vi "EMV T7 Flow Conditions.vi"(4 "Detection Slope":dbl=0.2 format="%#_13g", 7 "Mixing Valve.Flow State (0x4009)":u8, 8 "error in (no error)":errorcluster, 10 "T7_DELTA_FLOW_THRESHOLD":dbl, 11 "T7 History":dbl[](array[numeric])) -> (0 "error out":errorcluster, 1 "PI Detect?":bool, 2 "T7 Detect?":bool, 3 "Flow Detect?":bool)   [LabVIEW 2020]
panel:
  out "Slope Chart":dbl(graph)
  in  "T7_DELTA_INDICATING_FLOW":dbl
  in  "Cold Water Supply Temperature":dbl
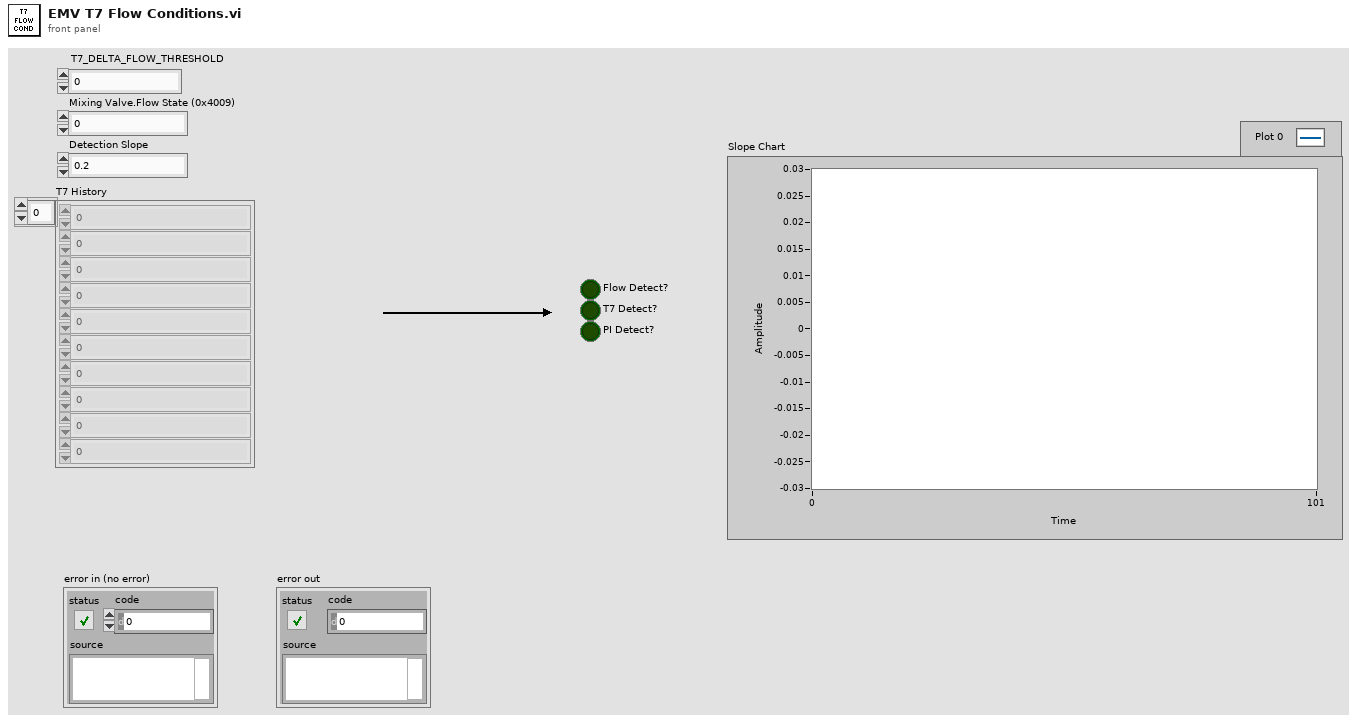
[diagram p1: front panel]
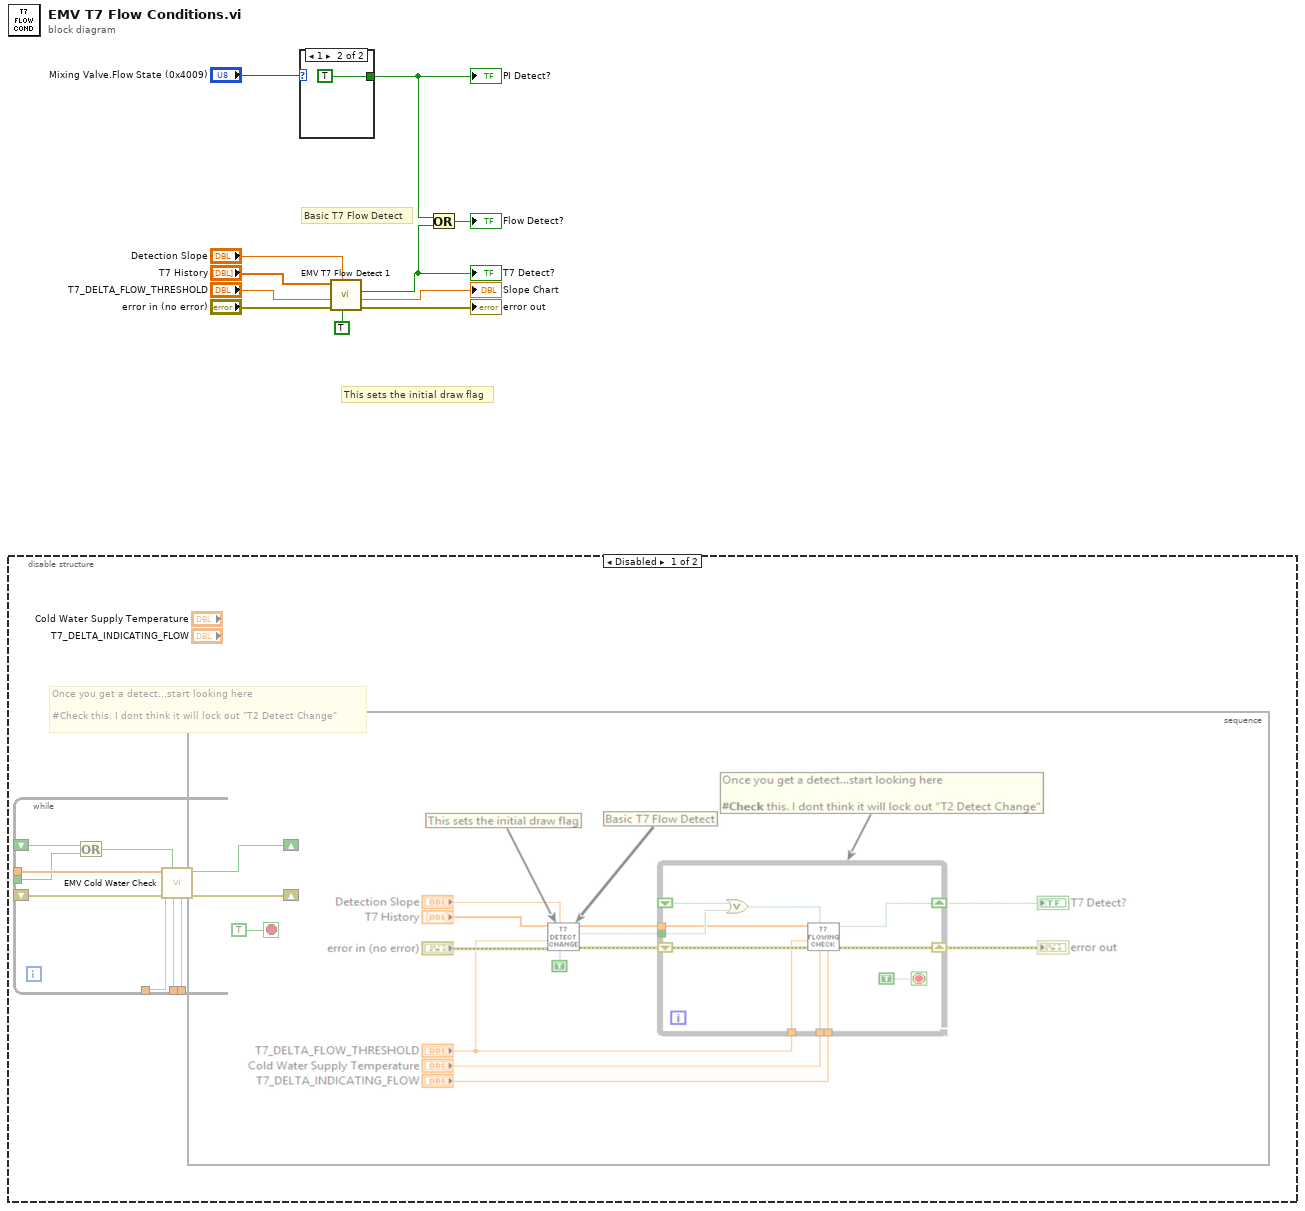
[diagram p0: block diagram]
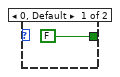
[diagram p2: hidden frame]
diagram:
  # "Basic T7 Flow Detect"
  # "This sets the initial draw flag"
  n1 = disable-structure shown="Disabled" {
    frame Disabled {
      # "Once you get a detect...start looking here\n\n#Check this. I dont think it will lock out \"T2 Detect Change\""
      n2 = while {
        tunnel: _ -> [w16]
        tunnel: _ -> [w22]
        tunnel: _ -> [w21]
        tunnel: _ -> [w18]
        shift-right: [w19] -> _
        shift-left: _ -> [w15]
        shift-right: [w20] -> _
        shift-left: _ -> [w14]
        tunnel: _ -> [w13]
        stop <- TRUE stop-if-true
        n3 = Or(x=w14, y=w13) -> (x .or. y?=w12:bool)
        n4 = call "EMV Cold Water Check.vi"("T7_DELTA_INDICATING_FLOW"=w22, "Cold Water Supply Temperature"=w21, "T7 Detect?"=w12, "error in (no error)"=w15, "T7_DELTA_FLOW_THRESHOLD"=w18, "Current T7 Temperatures"=w16) -> ("error out"=w19:errorcluster, "T7 Detect?"=w20:bool)  [unwired: 4 in]
      }
      n5 = stacked-sequence {
        frame #0 {
        }
      }
    }
    frame Enabled {
    }
  }
  n6 = case shown="1" "Mixing Valve.Flow State (0x4009)" {
    tunnel: [FALSE TRUE] -> w2
    frame 0, Default {
    }
    frame 1 {
    }
  }
  "PI Detect?" <- w2
  n7 = call "EMV T7 Flow Detect 1.vi"("Detect Flow Start?"=TRUE, "Detection Slope"="Detection Slope", "error in (no error)"="error in (no error)", "T7_DELTA_FLOW_THRESHOLD"="T7_DELTA_FLOW_THRESHOLD", "Current T7 Temperatures"="T7 History") -> ("error out"=→"error out":errorcluster, "slope"=→"Slope Chart":dbl, "Detection?"=w3:bool)  [unwired: 3 in, 1 out]
  "T7 Detect?" <- w3
  n8 = Or(x=w2, y=w3) -> (x .or. y?=→"Flow Detect?":bool)
